vi "Three Button Dialog w. Icon.vi"(4 "Allow User to Close Dialog (T)":bool=TRUE, 5 "Text.Justification":enum16{"Left", "Center", "Right"}(ring), 6 "Toggle Key Shortcut (<Return>, , <Esc>":T2(array[cluster])=[{"Focus"=FALSE, "Control"=FALSE, "Shift"=FALSE, "Key"="<Return>"}, {"Focus"=FALSE, "Control"=FALSE, "Shift"=FALSE, "Key"=""}, {"Focus"=FALSE, "Control"=FALSE, "Shift"=FALSE, "Key"="<Escape>"}], 7 "Window Title (\"\")":string, 9 "Symbol":T1, 10 "Button Strings":string[](array[string])=["Yes", "No", "Cancel"], 11 "Message":string) -> (3 "Which Button?":T3=enum."Center Button")   [LabVIEW 2013, in "Workspace MultiY Graph.lvlib" / "Alert Dialogs.lvlib"]
uses:
  Alert Dialogs.lvlib
  Dlg Symbol Picture.ctl
  Dlg Button.ctl
  Dlg Symbol.ctl
  Dlg State.ctl
  <vilib>/Utility/miscctls.llb/LVPointTypeDef.ctl
  <vilib>/Utility/miscctls.llb/LVBoundsTypeDef.ctl
panel:
  out "Symbol Display":T4
  out "error out":errorcluster
  out "Message Display":string
  in  "Right Button":bool
  in  "Center Button":bool
  in  "Left Button":bool
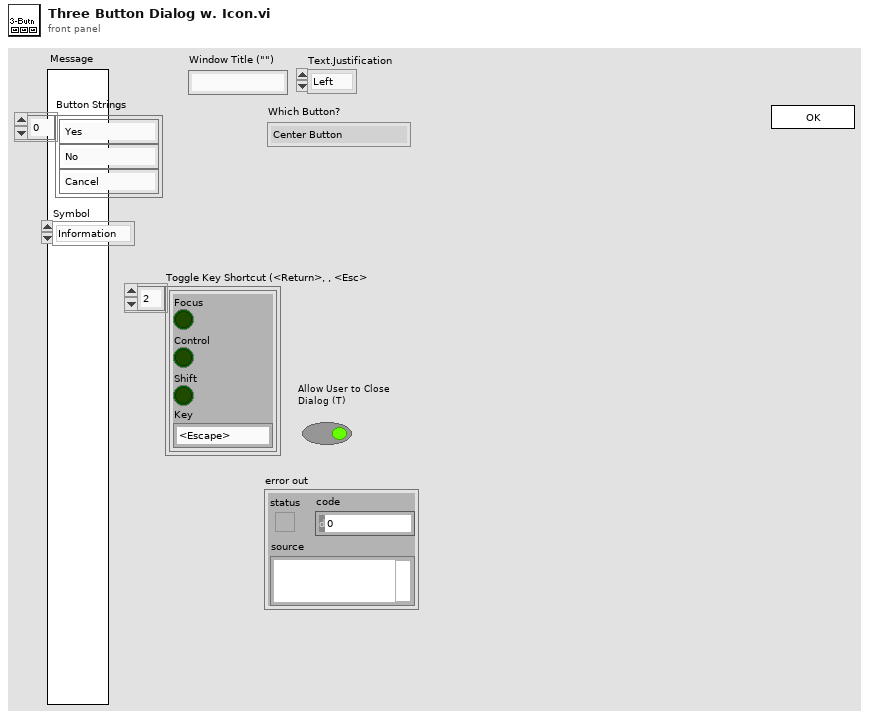
[diagram p1: front panel]
types:
  T1 = typedef "Workspace MultiY Graph.lvlib/Alert Dialogs.lvlib/Dlg Symbol.ctl" = enum16{"Information", "Help", "Warning", "Error"}
  T2 = cluster{"Focus":bool, "Control":bool, "Shift":bool, "Key":string}[]
  T3 = typedef "Workspace MultiY Graph.lvlib/Alert Dialogs.lvlib/Dlg Button.ctl" = enum16{"Left Button", "Center Button", "Right Button", "Window Close"}
  T4 = typedef "Workspace MultiY Graph.lvlib/Alert Dialogs.lvlib/Dlg Symbol Picture.ctl" = u16
  T5 = typedef "Workspace MultiY Graph.lvlib/Alert Dialogs.lvlib/Dlg State.ctl" = enum16{"Initialize", "Set Values", "Resize Controls", "Move Buttons", "Resize Panel", "Do UI"}
  T6 = typedef "LVPointTypeDef.ctl" = cluster{"Horizontal":i16, "Vertical":i16}
  T7 = typedef "LVBoundsTypeDef.ctl" = cluster{"Width":u32, "Height":u32}
  T8 = cluster{"Focus":bool, "Control":bool, "Shift":bool, "Key":string}
  T9 = typedef "LVPositionTypeDef.ctl" = cluster{"Left":i32, "Top":i32}
  T10 = typedef "LVRectTypeDef.ctl" = cluster{"Left":i16, "Top":i16, "Right":i16, "Bottom":i16}
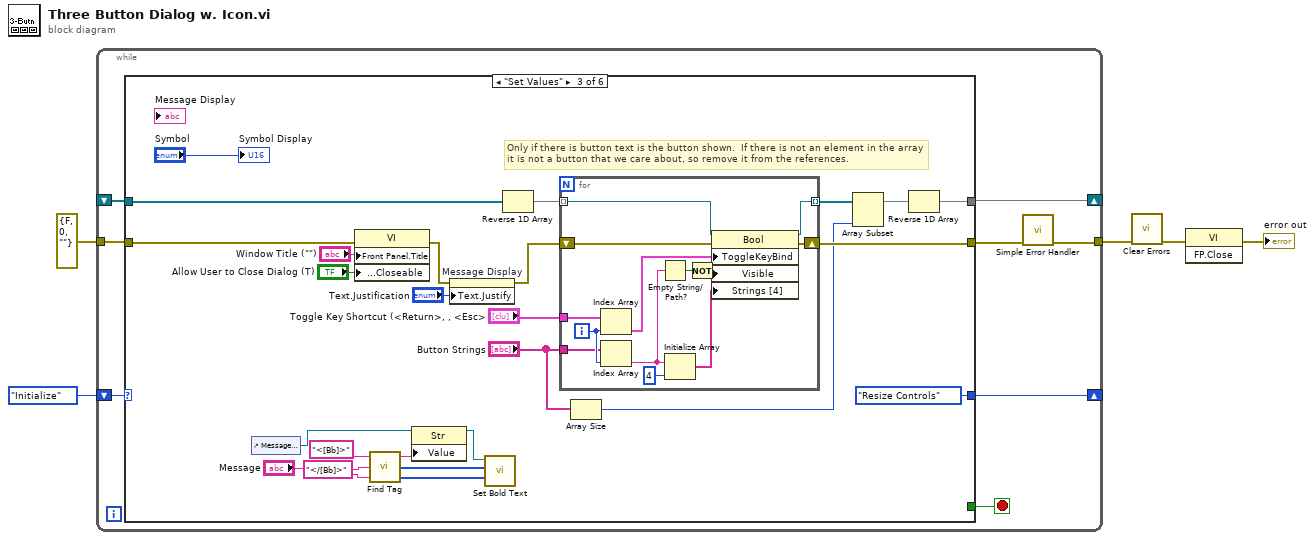
[diagram p0: block diagram]
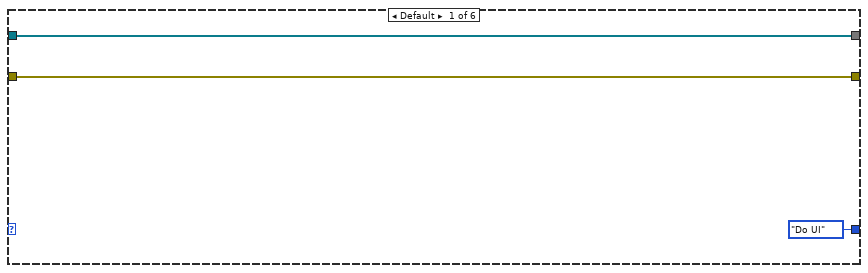
[diagram p2: hidden frame]
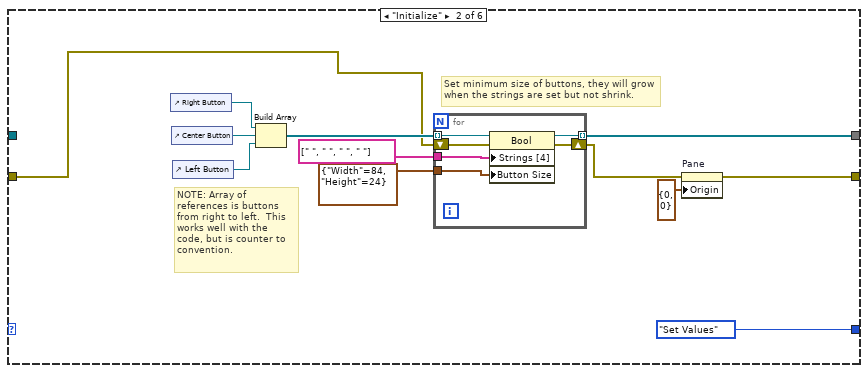
[diagram p3: hidden frame]
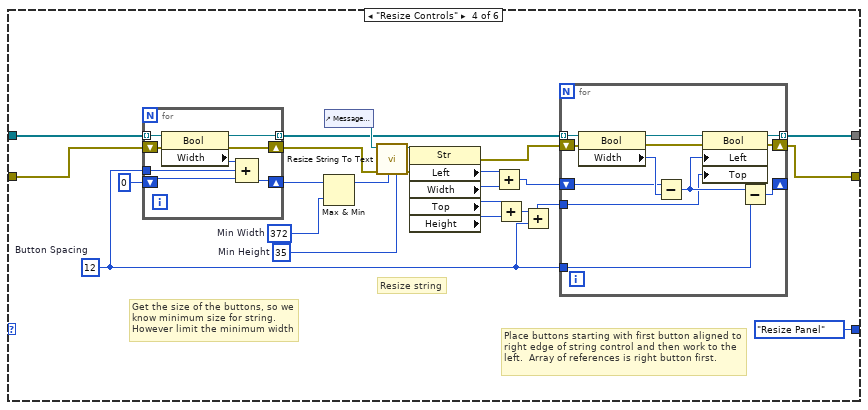
[diagram p4: hidden frame]
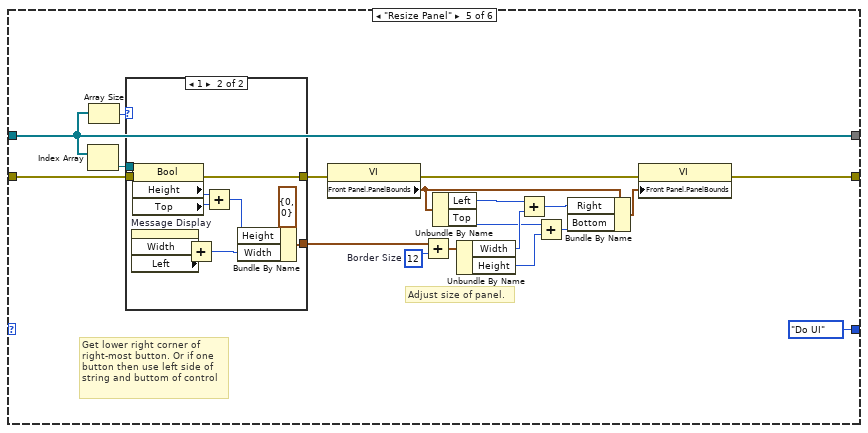
[diagram p5: hidden frame]
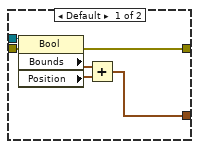
[diagram p6: hidden frame]
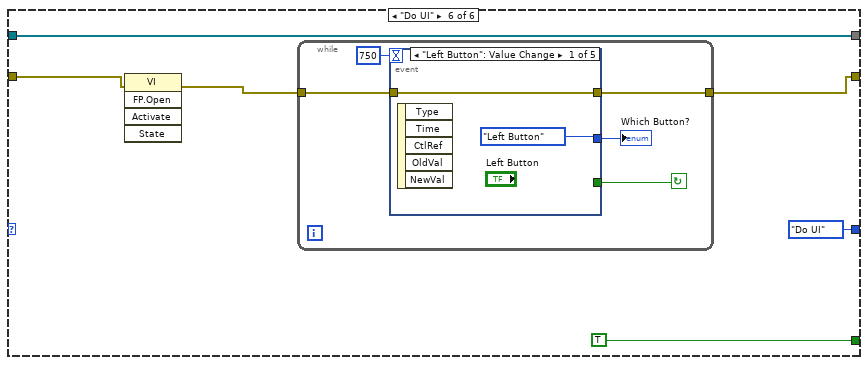
[diagram p7: hidden frame]
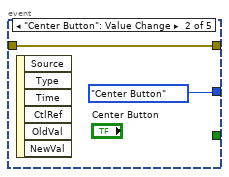
[diagram p8: hidden frame]
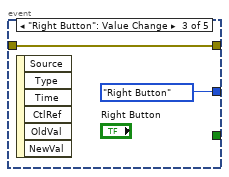
[diagram p9: hidden frame]
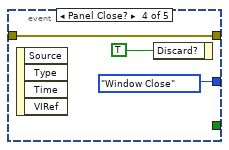
[diagram p10: hidden frame]
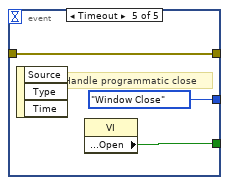
[diagram p11: hidden frame]
diagram:
  n1 = while {
    shift-right: [w7] -> _
    shift-left: Dlg_State."Initialize" ("sit Dialog Stage") -> [w12]
    shift-right: [w8] -> _
    shift-left: _ -> [w11]
    tunnel: errorcluster {"status"=FALSE, "code"=0, "source"=""} ("error out") -> [w9]
    tunnel: [w6] -> w3
    stop <- w13 stop-if-true
    n2 = case shown="\"Set Values\"" w12 {
      tunnel: [_ _ _ _ _ TRUE] -> w13
      tunnel: w11 -> [w16 _ w50 w83 w119 w157]
      tunnel: [w15 w18 w51 w79 w121 w155] -> w10
      tunnel: w9 -> [w15 w17 w52 w82 w123 w154]
      tunnel: [w16 w26 w47 w80 w119 w157] -> w8
      tunnel: [Dlg_State."Do UI" ("sit Dialog Stage") Dlg_State."Set Values" ("sit Dialog Stage") Dlg_State."Resize Controls" ("sit Dialog Stage") Dlg_State."Resize Panel" ("sit Dialog Stage") Dlg_State."Do UI" ("sit Dialog Stage") Dlg_State."Do UI" ("sit Dialog Stage")] -> w7
      frame Default {
      }
      frame "Initialize" {
        # "NOTE: Array of references is buttons from right to left.  This works well with the code, but is counter to convention."
        # "Set minimum size of buttons, they will grow when the strings are set but not shrink."
        n3 = control-ref of="Right Button"() -> (w22:refnum<vi>)
        n4 = control-ref of="Center Button"() -> (w28:refnum<vi>)
        n5 = control-ref of="Left Button"() -> (w21:refnum<vi>)
        n6 = Build Array(w22, w28, w21) -> (w27:refnum<vi>[])
        n7 = for {
          tunnel: w27 -> [w34] mode=indexing
          tunnel: [w33] -> w26 mode=indexing
          tunnel: string[] [" ", " ", " ", " "] ("Strings [4]") -> [w32]
          tunnel: cluster{"Width":u32, "Height":u32} {"Width"=84, "Height"=24} ("Button Size") -> [w31]
          shift-right: [w29] -> w19
          shift-left: w17 -> [w30]
          n8 = property on="Property Node" class="Bool"(reference=w34, error in=w30, "Strings [4]"=w32, "Button Size"=w31) -> (reference out=w33:refnum<vi>, error out=w29:errorcluster)
        }
        n9 = property on="Pane" class="Pane"(error in=w19, "Origin"=T6 {"Horizontal"=0, "Vertical"=0}) -> (error out=w18:errorcluster)  [unwired: 1 in, 1 out]
      }
      frame "Set Values" {
        # "Only if there is button text is the button shown.  If there is not an element in the array it is not a button that we care about, so remove it from the references."
        n10 = control-ref of="Message Display"() -> (w36:refnum<vi>)
        n11 = property class="VI"(error in=w52, "Front Panel.Title"="Window Title (\"\")", "Front Panel.Closeable"="Allow User to Close Dialog (T)") -> (error out=w55:errorcluster)  [unwired: 1 in, 1 out]
        n12 = call <vilib>:"Find Tag.vi"("string"="Message", "close tag"="</[Bb]>" ("don't translate!"), "open tag"="<[Bb]>" ("don't translate!")) -> ("Length"=w38:i32[], "Start"=w39:i32[], "string out"=w40:string)
        n13 = property on="Property Node" class="Str"(reference=w36, "Value"=w40) -> (reference out=w35:refnum<vi>)  [unwired: 1 in, 1 out]
        n14 = property on="Message Display" class="Str"(error in=w55, "Text.Justify"="Text.Justification") -> (error out=w54:errorcluster)  [unwired: 1 in, 1 out]
        n15 = call <vilib>:"Set Bold Text.vi"("Length"=w38, "Start"=w39, "text"=w35) -> ()  [unwired: 1 in, 3 out]
        n16 = Reverse 1D Array(array=w50) -> (reversed array=w48:refnum<vi>[])
        n17 = for {
          tunnel: "Button Strings" -> [w64]
          tunnel: "Toggle Key Shortcut (<Return>, , <Esc>" -> [w71]
          shift-right: [w70] -> w51
          shift-left: w54 -> [w69]
          tunnel: w48 -> [w68] mode=indexing
          tunnel: [w66] -> w44 mode=indexing
          i -> [w65]
          n18 = Index Array(array=w71, index=w65) -> (element=w67:T8)
          n19 = Index Array(array=w64, index=w65) -> (element=w63:string)
          n20 = Empty String/Path?(string/path=w63) -> (empty?=w61:bool)
          n21 = Initialize Array(w63, 4 ("dimension size")) -> (w62:string[])
          n22 = Not(x=w61) -> (.not. x?=w60:bool)
          n23 = property on="Property Node" class="Bool"(reference=w68, error in=w69, "ToggleKeyBind"=w67, "Visible"=w60, "Strings [4]"=w62) -> (reference out=w66:refnum<vi>, error out=w70:errorcluster)
        }
        n24 = Array Size(array="Button Strings") -> (size(s)=w43:i32)
        n25 = Array Subset(array=w44, length=w43) -> (w45:refnum<vi>[])  [unwired: 1 in]
        n26 = Reverse 1D Array(array=w45) -> (reversed array=w47:refnum<vi>[])
        "Symbol Display" <- "Symbol"
      }
      frame "Resize Controls" {
        w77 = u32 372  # Min Width
        w84 = u32 12  # Button Spacing
        w96 = u32 35  # Min Height
        # "Place buttons starting with first button aligned to right edge of string control and then work to the left.  Array of references is right button first."
        # "Resize string"
        # "Get the size of the buttons, so we know minimum size for string.  However limit the minimum width"
        n27 = for {
          tunnel: w83 -> [w116] mode=indexing
          tunnel: w84 -> [w114]
          shift-right: [w113] -> w93
          shift-left: u32 0 -> [w112]
          shift-right: [w110] -> w92
          shift-left: w82 -> [w111]
          tunnel: [w109] -> w76 mode=indexing
          n28 = property class="Bool"(reference=w116, error in=w111) -> (reference out=w109:refnum<vi>, error out=w110:errorcluster, "Width"=w115:u32)
          n29 = Compound Arithmetic op=ADD(w115, w114, w112) -> (w113:u32)
        }
        n30 = Max & Min(x=w93, y=w77) -> (max(x,y)=w78:u32)  [unwired: 1 out]
        n31 = control-ref of="Message Display"() -> (w95:refnum<vi>)
        n32 = call "Resize String To Text.vi"("Min Height"=w96, "Min Width"=w78, "error in (no error)"=w92, "String Ref"=w95) -> ("error out"=w90:errorcluster, "dup String Ref"=w91:refnum<vi>)  [unwired: 2 in, 4 out]
        n33 = property class="Str"(reference=w91, error in=w90) -> (error out=w87:errorcluster, "Left"=w89:i32, "Width"=w88:u32, "Top"=w86:i32, "Height"=w85:u32)  [unwired: 1 out]
        n34 = Add(x=w89, y=w88) -> (x+y=w75:u32)
        n35 = Add(x=w86, y=w85) -> (x+y=w74:u32)
        n36 = Add(x=w74, y=w84) -> (x+y=w73:u32)
        n37 = for {
          tunnel: w76 -> [w108] mode=indexing
          shift-right: [w101] -> _
          shift-left: w75 -> [w106]
          tunnel: w84 -> [w105]
          shift-right: [w99] -> w79
          shift-left: w87 -> [w100]
          tunnel: w73 -> [w98]
          tunnel: [w97] -> w80 mode=indexing
          n38 = property class="Bool"(reference=w108, error in=w100) -> (reference out=w104:refnum<vi>, error out=w103:errorcluster, "Width"=w107:u32)
          n39 = Subtract(x=w106, y=w107) -> (x-y=w102:u32)
          n40 = property class="Bool"(reference=w104, error in=w103, "Left"=w102, "Top"=w98) -> (reference out=w97:refnum<vi>, error out=w99:errorcluster)
          n41 = Subtract(x=w102, y=w105) -> (x-y=w101:u32)
        }
      }
      frame "Resize Panel" {
        w118 = u32 12  # Border Size
        # "Adjust size of panel."
        # "Get lower right corner of right-most button. Or if one button then use left side of string and buttom of control"
        n42 = Index Array(array=w119) -> (element=w124:refnum<vi>)  [unwired: 1 in]
        n43 = Array Size(array=w119) -> (size(s)=w117:i32)
        n44 = case shown="1" w117 {
          tunnel: [w139 w145] -> w135
          tunnel: w124 -> [w138 w150]
          tunnel: w123 -> [w137 w149]
          tunnel: [w136 w148] -> w122
          frame Default {
            n45 = property class="Bool"(reference=w138, error in=w137) -> (error out=w136:errorcluster, "Bounds"=w141:T7, "Position"=w140:T9)  [unwired: 1 out]
            n46 = Add(x=w141, y=w140) -> (x+y=w139:T7)
          }
          frame 1 {
            n47 = property on="Message Display" class="Str"() -> ("Width"=w146:u32, "Left"=w147:i32)  [unwired: 2 in, 2 out]
            n48 = property class="Bool"(reference=w150, error in=w149) -> (error out=w148:errorcluster, "Height"=w152:u32, "Top"=w151:i32)  [unwired: 1 out]
            n49 = Add(x=w146, y=w147) -> (x+y=w143:u32)
            n50 = Add(x=w152, y=w151) -> (x+y=w142:u32)
            n51 = Bundle By Name(cluster=T7 {"Width"=0, "Height"=0} ("Bounds"), "Height"=w142, "Width"=w143) -> (w145:T7)
          }
        }
        n52 = property class="VI"(error in=w122) -> (error out=w125:errorcluster, "Front Panel.PanelBounds"=w128:T10)  [unwired: 1 in, 1 out]
        n53 = Add(x=w135, y=w118) -> (x+y=w134:T7)
        n54 = Unbundle By Name(w128) -> ("Left"=w133:i16, "Top"=w131:i16)
        n55 = Unbundle By Name(w134) -> ("Width"=w132:u32, "Height"=w130:u32)
        n56 = Add(x=w133, y=w132) -> (x+y=w129:u32)
        n57 = Add(x=w131, y=w130) -> (x+y=w127:u32)
        n58 = Bundle By Name(cluster=w128, "Right"=w129, "Bottom"=w127) -> (w126:T10)
        n59 = property class="VI"(error in=w125, "Front Panel.PanelBounds"=w126) -> (error out=w121:errorcluster)  [unwired: 1 in, 1 out]
      }
      frame "Do UI" {
        n60 = invoke class="VI" method="FP.Open"(error in=w154) -> (error out=w153:errorcluster)  [unwired: 4 in, 4 out]
        n61 = while {
          tunnel: [w162] -> w155
          tunnel: w153 -> [w161]
          stop <- w160 continue-if-true
          n62 = event shown="[0] \"Left Button\": Value Change" {
            selector: _ -> [_ _ _ _ _]
            dyn-events: _ -> [_ _ _ _ _]
            timeout: 750 -> [_ _ _ _ _]
            tunnel: [Dlg_Button."Left Button" ("Which Button?") Dlg_Button."Center Button" ("Which Button?") Dlg_Button."Right Button" ("Which Button?") Dlg_Button."Window Close" ("Which Button?") Dlg_Button."Window Close" ("Which Button?")] -> w163
            tunnel: w161 -> [w165 w167 w169 w172 w174]
            tunnel: [w165 w167 w169 w172 w174] -> w162
            tunnel: [_ _ _ _ w175] -> w160
            event "Left Button": Value Change {
              n63 = event-data() -> ()  [unwired: 6 out]
            }
            event "Center Button": Value Change {
              n64 = event-data() -> ()  [unwired: 7 out]
            }
            event "Right Button": Value Change {
              n65 = event-data() -> ()  [unwired: 7 out]
            }
            event Panel Close? {
              n66 = event-data() -> ()  [unwired: 5 out]
              n67 = event-data("Discard?"=TRUE) -> ()  [unwired: 1 in, 1 out]
            }
            event Timeout {
              # "Handle programmatic close"
              n68 = event-data() -> ()  [unwired: 4 out]
              n69 = property class="VI"() -> ("Front Panel Window:Open"=w175:bool)  [unwired: 2 in, 2 out]
            }
          }
          "Which Button?" <- w163
        }
      }
    }
    n70 = call <vilib>:"Simple Error Handler.vi"("error in (no error)"=w10) -> ("error out"=w6:errorcluster)  [unwired: 1 in, 7 out]
  }
  n71 = call <vilib>:"Clear Errors.vi"("error in (no error)"=w3) -> ("error out"=w1:errorcluster)  [unwired: 6 out]
  n72 = invoke class="VI" method="FP.Close"(error in=w1) -> (error out=→"error out":errorcluster)  [unwired: 2 in, 2 out]
